vi "队列采集显示.vi"() -> ()   [LabVIEW 2011]
panel:
  in  "stop":bool
  out "Waveform Chart":dbl(graph)
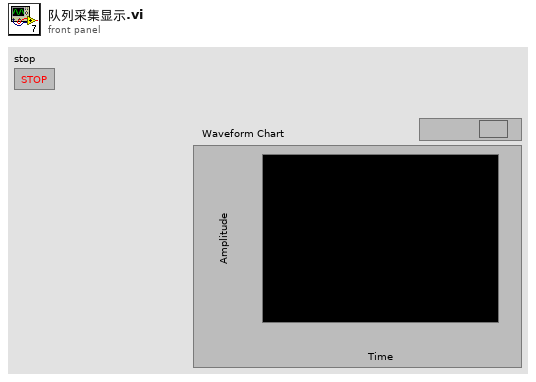
[diagram p1: front panel]
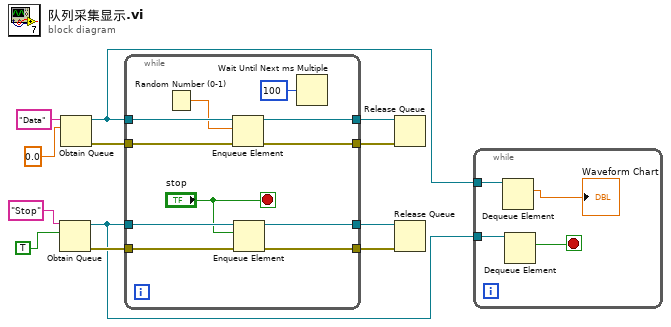
[diagram p0: block diagram]
diagram:
  n1 = Obtain Queue(name (unnamed)="Stop", element data type=TRUE) -> (queue out=w1:refnum<queue>, error out=w5:errorcluster)  [unwired: 3 in, 1 out]
  n2 = Obtain Queue(name (unnamed)="Data", element data type=0.0) -> (queue out=w2:refnum<queue>, error out=w11:errorcluster)  [unwired: 3 in, 1 out]
  n3 = while {
    tunnel: w2 -> [w23]
    tunnel: [w22] -> w12
    tunnel: w11 -> [w21]
    tunnel: [w20] -> w10
    tunnel: w1 -> [w19]
    tunnel: w5 -> [w18]
    tunnel: [w17] -> w4
    tunnel: [w16] -> w3
    stop <- "stop" stop-if-true
    n4 = Random Number (0-1)() -> (number: 0 to 1=w14:dbl)
    n5 = Enqueue Element(queue=w23, element=w14, error in (no error)=w21) -> (queue out=w22:refnum<queue>, error out=w20:errorcluster)  [unwired: 1 in, 1 out]
    n6 = Enqueue Element(queue=w19, element="stop", error in (no error)=w18) -> (queue out=w17:refnum<queue>, error out=w16:errorcluster)  [unwired: 1 in, 1 out]
    n7 = Wait Until Next ms Multiple(millisecond multiple=u32 100) -> ()  [unwired: 1 out]
  }
  n8 = Release Queue(queue=w12, error in (no error)=w10) -> ()  [unwired: 1 in, 3 out]
  n9 = Release Queue(queue=w4, error in (no error)=w3) -> ()  [unwired: 1 in, 3 out]
  n10 = while {
    tunnel: w2 -> [w27]
    tunnel: w1 -> [w26]
    stop <- w24 stop-if-true
    n11 = Dequeue Element(queue=w27) -> (element=→"Waveform Chart":dbl)  [unwired: 2 in, 3 out]
    n12 = Dequeue Element(queue=w26) -> (element=w24:bool)  [unwired: 2 in, 3 out]
  }
